vi "GetQY.vi"(2 "error in":errorcluster) -> (0 "error out":errorcluster, 1 "data":string)   [LabVIEW 2010]
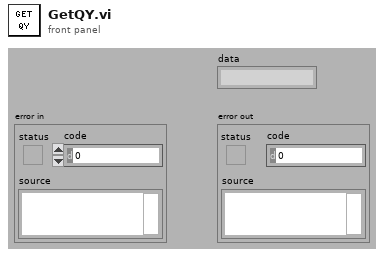
[diagram p1: front panel]
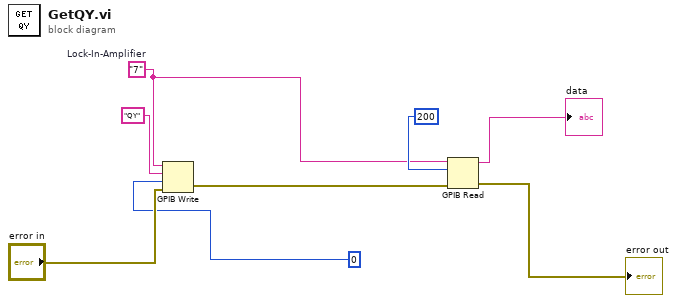
[diagram p0: block diagram]
diagram:
  w3 = "7"  # Lock-In-Amplifier
  n1 = GPIB Write(0:w3, 1:"QY", 2:i16 0 ("mode (0)"), 3:"error in") -> (6:w2:errorcluster)  [unwired: 1 in, 1 out]
  n2 = GPIB Read(0:w3, 1:200, 3:w2) -> (5:→"data":string, 7:→"error out":errorcluster)  [unwired: 2 in, 1 out]
